vi "Running Min.vi"(3 "Starting Min":u32=4294967295, 6 "Reset":bool, 7 "Next Value":u32) -> (1 "Running Min":u32)   [LabVIEW 2016]
doc: "This SubVI keeps a running min value based on the input value and a starting min value. The current running min is resetable."
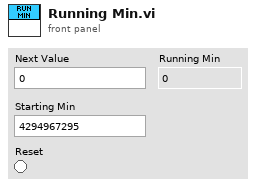
[diagram p1: front panel]
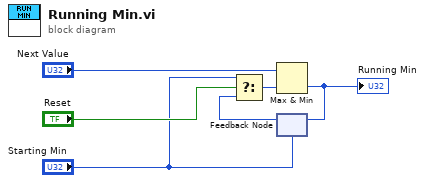
[diagram p0: block diagram]
diagram:
  n1 = feedback #1("Starting Min") -> (w3:u32)
  n2 = Select(t="Starting Min", s="Reset", f=w3) -> (s? t:f=w2:u32)
  n3 = Max & Min(x="Next Value", y=w2) -> (min(x,y)=w1:u32)  [unwired: 1 out]
  "Running Min" <- w1
  n4 = feedback-in #1(w1) -> ()
